vi "KE622x -- Get List Sweep Params.vi"(0 "Resource In":refnum<visa-resource-name>, 1 "Check For SCPI Errors? (T)":bool=TRUE, 11 "error in (no error)":errorcluster) -> (4 "Resource Out (dupl)":refnum<visa-resource-name>, 8 "List Sweep Params":T1 {"List Sweep Steps"."Current Level (A)" min=-0.105 max=0.105 format="%.4p"; "List Sweep Steps"."Source Delay (s)" min=0.001 max=1000.0 step=0.001 format="%.3f"; "List Sweep Steps"."Voltage Limit (V)" min=0.1 max=105.0 step=0.01 format="%.2p"}, 15 "error out":errorcluster)   [LabVIEW 2010, in "Keithley 622x.lvlib"]
doc: "Returns the individual points in a list current sweep and also whether or not the list current sweep will abort on a compliance (voltage limit) condition."
uses:
  Keithley 622x.lvlib
  Typedefs/KE622x -- List Sweep Params.ctl
  Typedefs/KE622x -- List Sweep Steps.ctl
  Typedefs/KE622x -- List Sweep Step.ctl
  Typedefs/KE622x -- Current Level.ctl
  Typedefs/KE622x -- Source Delay.ctl
  Typedefs/KE622x -- Voltage Limit.ctl
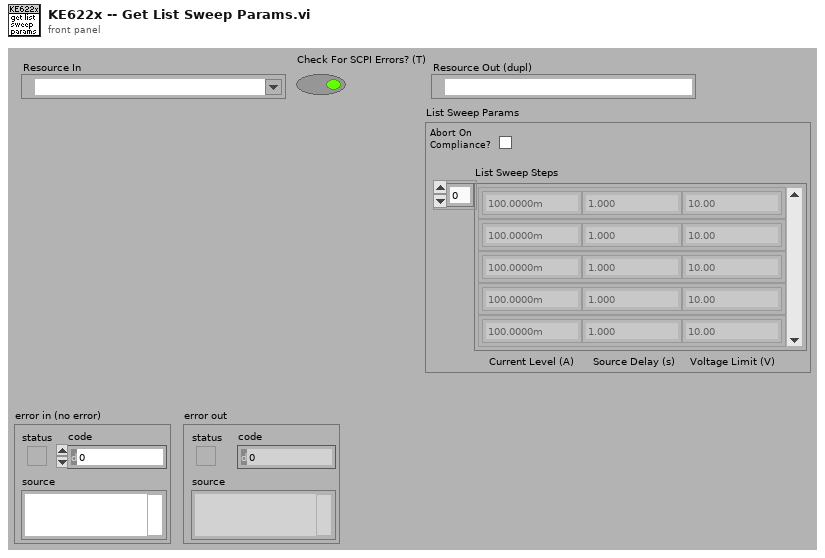
[diagram p1: front panel]
types:
  T1 = typedef "Keithley 622x.lvlib/KE622x -- List Sweep Params.ctl" = cluster{"Abort On\nCompliance?":bool, "List Sweep Steps":T2}
  T2 = typedef "Keithley 622x.lvlib/KE622x -- List Sweep Steps.ctl" = T3[]
  T3 = typedef "Keithley 622x.lvlib/KE622x -- List Sweep Step.ctl" = cluster{"Current Level (A)":T4, "Source Delay (s)":T5, "Voltage Limit (V)":T6}
  T4 = typedef "Keithley 622x.lvlib/KE622x -- Current Level.ctl" = dbl
  T5 = typedef "Keithley 622x.lvlib/KE622x -- Source Delay.ctl" = dbl
  T6 = typedef "Keithley 622x.lvlib/KE622x -- Voltage Limit.ctl" = dbl
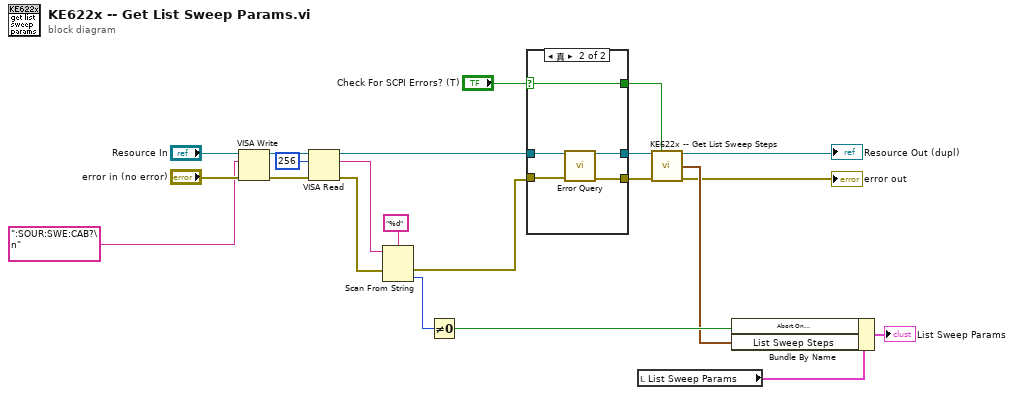
[diagram p0: block diagram]
diagram:
  n1 = VISA Write(VISA resource name="Resource In", write buffer=":SOUR:SWE:CAB?\n" ("format string"), error in (no error)="error in (no error)") -> (VISA resource name out=w18:refnum<visa-resource-name>, error out=w17:errorcluster)  [unwired: 1 out]
  n2 = VISA Read(VISA resource name=w18, byte count=u32 256, error in (no error)=w17) -> (VISA resource name out=w11:refnum<visa-resource-name>, read buffer=w13:string, error out=w15:errorcluster)  [unwired: 1 out]
  n3 = Scan From String(format string="%d", input string=w13, error in=w15) -> (error out=w12:errorcluster, output 1=w10:i32)  [unwired: 2 in, 2 out]
  n4 = Not Equal To 0?(x=w10) -> (x != 0?=w5:bool)
  n5 = case shown="真" "Check For SCPI Errors? (T)" {
    selector: "Check For SCPI Errors? (T)" -> [w23 w26]
    tunnel: w11 -> [w25 w30]
    tunnel: w12 -> [w24 w29]
    tunnel: [w24 w28] -> w8
    tunnel: [w25 w27] -> w9
    tunnel: [w23 w26] -> w7
    frame False {
    }
    frame True {
      n6 = call "Error Query.vi"("VISA Resource In"=w30, "error in (no error)"=w29) -> ("VISA Resource Out (dupl)"=w27:refnum<visa-resource-name>, "error out"=w28:errorcluster)  [unwired: 10 in, 2 out]
    }
  }
  n7 = local read "List Sweep Params"() -> (w6:T1)
  n8 = call "KE622x -- Get List Sweep Steps.vi"("Resource In"=w9, "Check For SCPI Errors? (T)"=w7, "error in (no error)"=w8) -> ("Resource Out (dupl)"=→"Resource Out (dupl)":refnum<visa-resource-name>, "List Sweep Steps"=w4:T2, "error out"=→"error out":errorcluster)  [unwired: 9 in, 1 out]
  n9 = Bundle By Name(cluster=w6, "Abort On\nCompliance?"=w5, "List Sweep Steps"=w4) -> (→"List Sweep Params":T1)
